vi "Read Measurement (Others).vi"(0 "VISA resource name":refnum<visa-resource-name>, 5 "Timeout (10000 ms)":i32=10000 format="%.0g", 7 "Read Option (0)":i32 format="%.0g", 11 "error in (no error)":errorcluster) -> (4 "VISA resource name out":refnum<visa-resource-name>, 6 "Measurement Data":dbl[](array[numeric]), 15 "error out":errorcluster)   [LabVIEW 2018, in "Agilent MXA Series.lvlib"]
doc: "Reads the measurement result from the spectrum analyzer (ACP, Burst Power, Spurious Emissions, Spectrum Emission Mask)"
uses:
  Agilent MXA Series.lvlib
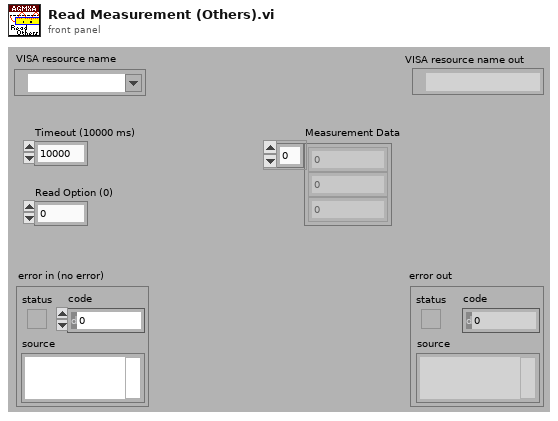
[diagram p1: front panel]
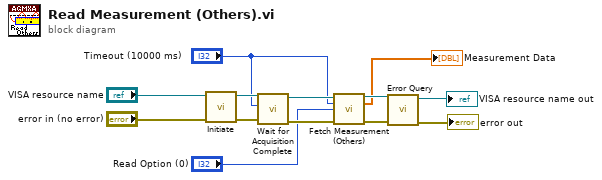
[diagram p0: block diagram]
diagram:
  n1 = call "Initiate.vi"("error in (no error)"="error in (no error)", "VISA resource name"="VISA resource name") -> ("error out"=w10:errorcluster, "VISA resource name out"=w11:refnum<visa-resource-name>)  [unwired: 8 in]
  n2 = call "Wait for Acquisition Complete.vi"("error in (no error)"=w10, "Maximum Time (10000)"="Timeout (10000 ms)", "VISA resource name"=w11) -> ("error out"=w8:errorcluster, "VISA resource name out"=w9:refnum<visa-resource-name>)  [unwired: 7 in]
  n3 = call "Fetch Measurement (Others).vi"("VISA resource name"=w9, "Timeout (10000 ms)"="Timeout (10000 ms)", "Fetch Option (0)"="Read Option (0)", "error in (no error)"=w8) -> ("VISA resource name out"=w6:refnum<visa-resource-name>, "Measurement Data"=→"Measurement Data":dbl[], "error out"=w5:errorcluster)  [unwired: 9 in]
  n4 = call "Error Query.vi"("error in (no error)"=w5, "VISA resource name"=w6) -> ("error out"=→"error out":errorcluster, "VISA resource name out"=→"VISA resource name out":refnum<visa-resource-name>)  [unwired: 6 in, 2 out]
